vi "Define Trigger.vi"(7 "Trigger (0: Input)":u16(ring) items=["Input", "Output"], 8 "error in (no error)":errorcluster, 9 "Trigger Line (1)":u32=1, 10 "Event Detector (0: None)":u16(ring) items=["None", "Source", "Delay", "Sense"], 11 "VISA resource name":refnum<visa-resource-name>) -> (0 "error out":errorcluster, 3 "VISA resource name out":refnum<visa-resource-name>)   [LabVIEW 2020, in "Keithley 24XX.lvlib"]
uses:
  Keithley 24XX.lvlib
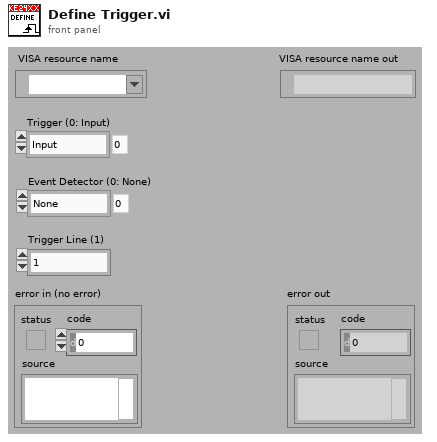
[diagram p1: front panel]
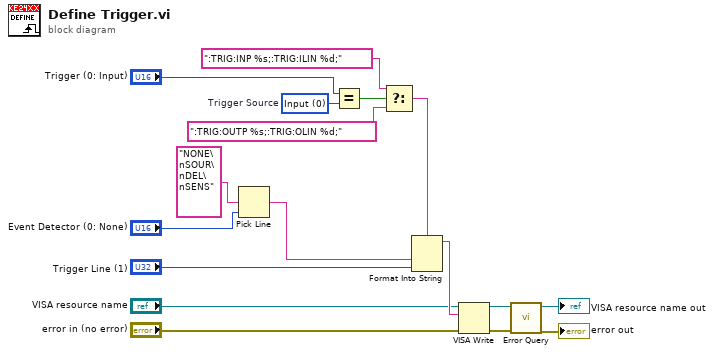
[diagram p0: block diagram]
diagram:
  w11 = u16 0 items=["Input", "Output"]  # Trigger Source
  n1 = Pick Line(multi-line string="NONE\nSOUR\nDEL\nSENS", line index="Event Detector (0: None)") -> (output string=w5:string)  [unwired: 1 in]
  n2 = Equal?(x="Trigger (0: Input)", y=w11) -> (x = y?=w7:bool)
  n3 = Select(t=":TRIG:INP %s;:TRIG:ILIN %d;", s=w7, f=":TRIG:OUTP %s;:TRIG:OLIN %d;") -> (s? t:f=w4:string)
  n4 = Format Into String(format string=w4, w5, "Trigger Line (1)") -> (resulting string=w3:string)  [unwired: 2 in, 1 out]
  n5 = VISA Write(VISA resource name="VISA resource name", write buffer=w3, error in (no error)="error in (no error)") -> (VISA resource name out=w14:refnum<visa-resource-name>, error out=w13:errorcluster)  [unwired: 1 out]
  n6 = call "Error Query.vi"("error in (no error)"=w13, "VISA resource name"=w14) -> ("error out"=→"error out":errorcluster, "VISA resource name out"=→"VISA resource name out":refnum<visa-resource-name>)  [unwired: 6 in, 2 out]
